vi "FTW-Scheduler-Destroy.vi"(1 "FTW Job Scheduler":refnum<class "FTW-Scheduler.lvclass">) -> (0 "Remaining Jobs":string)   [LabVIEW 2015, in "FTW-Scheduler.lvclass"]
uses:
  FTW-Scheduler.lvclass
  FTW-Scheduler.lvclass/FTW-Scheduler.ctl
panel:
  # "Inputs"
  # "Outputs"
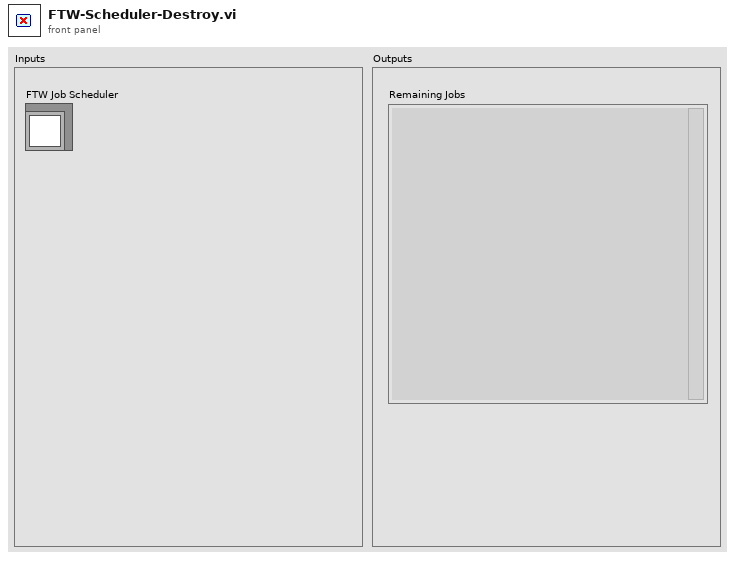
[diagram p1: front panel]
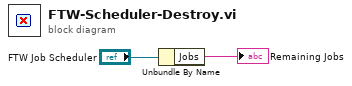
[diagram p0: block diagram]
diagram:
  n1 = Unbundle By Name("FTW Job Scheduler") -> ("Jobs"=→"Remaining Jobs":string)
